vi "FilterMetrics.vi"(11 "supported metrics":string[](array[string])) -> (2 "startup metrics supported in data viewer":string[](array[string]), 3 "high rate calculation supported metrics":string[](array[string]))   [LabVIEW 2017, in "McsaAnalysisHighRate.lvlib"]
uses:
  <vilib>/addons/InsightCM/Devices/Shared/Mcsa/McsaAnalysisHighRate/McsaAnalysisHighRate.lvlib
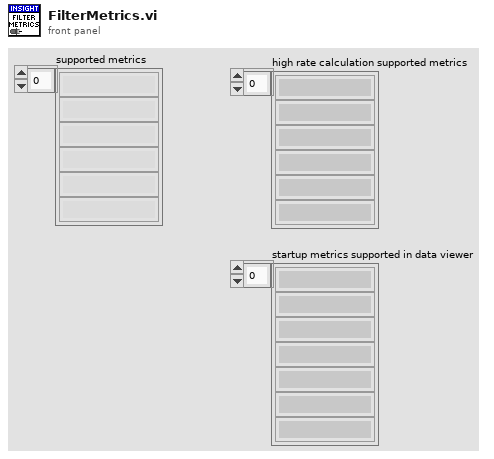
[diagram p1: front panel]
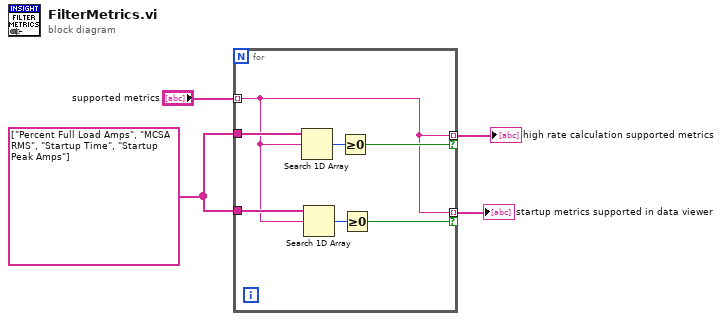
[diagram p0: block diagram]
diagram:
  w1 = string[] ["Percent Full Load Amps", "MCSA RMS", "Startup Time", "Startup Peak Amps"] ("value")
  n1 = for {
    tunnel: "supported metrics" -> [w5] mode=indexing
    tunnel: w1 -> [w11]
    tunnel: [w5] -> w3 mode=indexing if=w9
    tunnel: [w5] -> w2 mode=indexing if=w7
    tunnel: w1 -> [w6]
    n2 = Search 1D Array(1D array=w11, element=w5) -> (index of element=w10:i32)  [unwired: 1 in]
    n3 = Search 1D Array(1D array=w6, element=w5) -> (index of element=w8:i32)  [unwired: 1 in]
    n4 = Greater Or Equal To 0?(x=w10) -> (x >= 0?=w9:bool)
    n5 = Greater Or Equal To 0?(x=w8) -> (x >= 0?=w7:bool)
  }
  "high rate calculation supported metrics" <- w3
  "startup metrics supported in data viewer" <- w2
